vi "L14.vi"() -> ()   [LabVIEW 2012]
panel:
  out "output array":dbl[](array[numeric])
  out "max":i32
  out "Waveform Graph":i32[](graph)
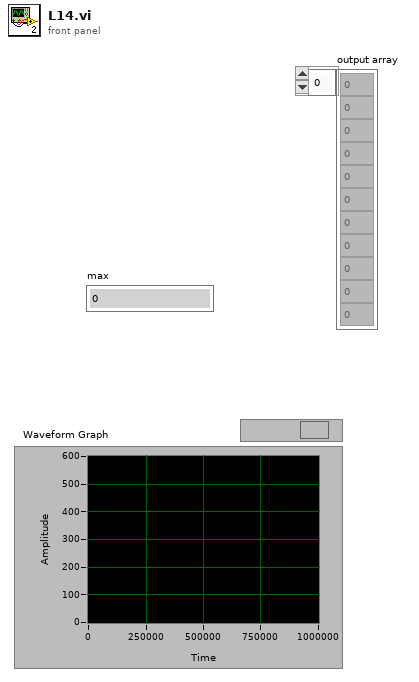
[diagram p1: front panel]
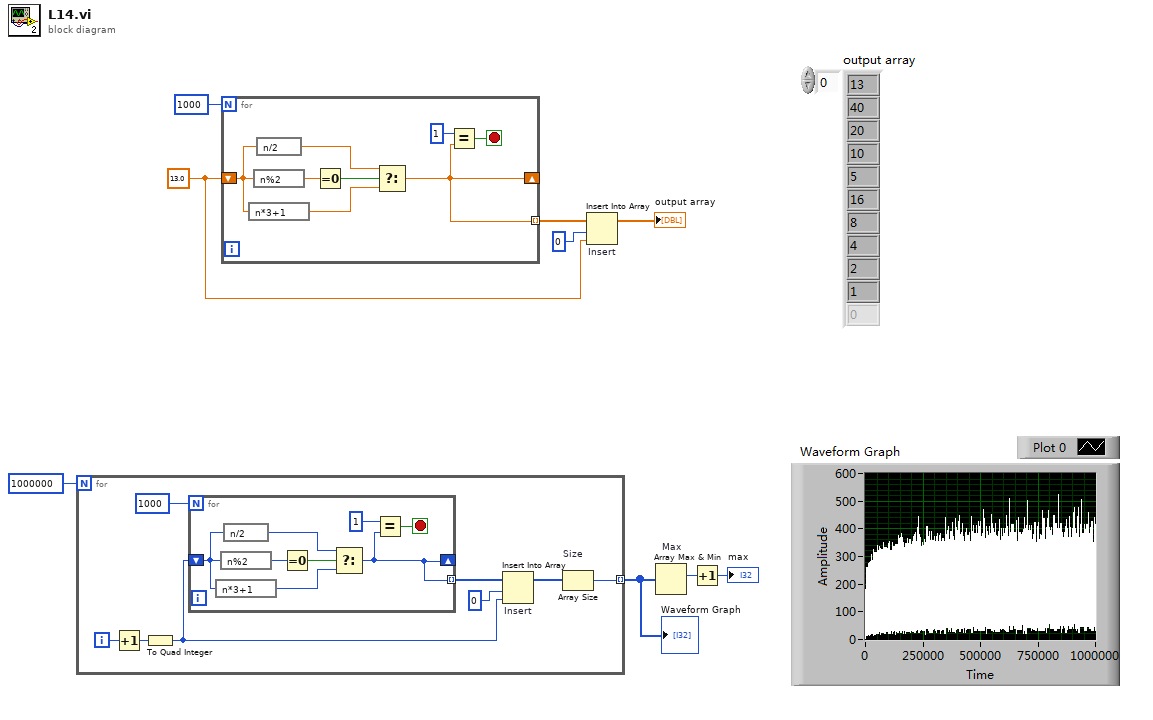
[diagram p0: block diagram]
diagram:
  w3 = 13.0
  n1 = for {
    N: 1000000 -> [_]
    tunnel: [w14] -> w8 mode=indexing
    i -> [w13]
    n2 = Increment(x=w13) -> (x+1=w12:i32)
    n3 = To Quad Integer(1:w12) -> (0:w11:i64)
    n4 = for {
      N: 1000 -> [_]
      shift-right: [w19] -> _
      shift-left: w11 -> [w21]
      tunnel: [w19] -> w17 mode=indexing
      stop <- w20 stop-if-true
      n5 = expression code="n*3+1"(w21) -> (w22:i64)
      n6 = expression code="n%2"(w21) -> (w25:i64)
      n7 = expression code="n/2"(w21) -> (w23:i64)
      n8 = Equal To 0?(x=w25) -> (x = 0?=w24:bool)
      n9 = Select(t=w23, s=w24, f=w22) -> (s? t:f=w19:i64)
      n10 = Equal?(x=i64 1 ("y"), y=w19) -> (x = y?=w20:bool)
    }
    n11 = Insert Into Array "Insert"(array=w17, index=0, new element=w11) -> (w15:i64[])
    n12 = Array Size "Size"(array=w15) -> (size(s)=w14:i32)
  }
  "Waveform Graph" <- w8
  n13 = for {
    N: 1000 -> [_]
    shift-right: [w27] -> _
    shift-left: w3 -> [w29]
    tunnel: [w27] -> w4 mode=indexing
    stop <- w28 stop-if-true
    n14 = expression code="n*3+1"(w29) -> (w30:dbl)
    n15 = expression code="n%2"(w29) -> (w33:dbl)
    n16 = expression code="n/2"(w29) -> (w31:dbl)
    n17 = Equal To 0?(x=w33) -> (x = 0?=w32:bool)
    n18 = Select(t=w31, s=w32, f=w30) -> (s? t:f=w27:dbl)
    n19 = Equal?(x=i64 1 ("y"), y=w27) -> (x = y?=w28:bool)
  }
  n20 = Insert Into Array "Insert"(array=w4, index=0, new element=w3) -> (→"output array":dbl[])
  n21 = Array Max & Min "Max"(array=w8) -> (max index (indices)=w7:i32)  [unwired: 3 out]
  n22 = Increment(x=w7) -> (x+1=→"max":i32)
